vi "cluster_v30.vi"() -> ()   [LabVIEW 2009]
panel:
  in  "stop":bool
  out "Waveform Graph":dbl[](graph)=[1.340619718021982, -0.6009860791806715, -0.0535520537195435, -0.009542246662558042, -0.0025019088903811522, -0.0008379211165242679, -0.00033229836709205973, -0.0001491346742136413, -7.356383530775908e-05, -3.9094873850847784e-05, -2.2068047028342232e-05, -1.3092803157888074e-05, -8.099534476939332e-06, -5.1922069190088255e-06, -3.4322006682237186e-06, -2.3302383349082557e-06, -1.6196706723518948e-06, -1.1494371287666694e-06, -8.309954579634783e-07, -6.108580258527588e-07, -4.55831665919915e-07, -3.448134329849513e-07, -2.6409078418298253e-07, -2.0457511909595536e-07, -1.601327682386241e-07, -1.265552528967856e-07, -1.0091080697079654e-07, -8.112824407953131e-08, -6.572525460615341e-08, -5.362814023445084e-08, -4.40504248915006e-08, -3.6409976192492306e-08, -3.0271687098320935e-08, -2.5307355322970933e-08, -2.126728244966514e-08, -1.7959955674597112e-08, -1.5237366748646937e-08, -1.298430431167563e-08, -1.111047491101763e-08, -9.544656805788532e-09, -8.230327650586232e-09, -7.122369864548406e-09, -6.184570317657947e-09, -5.387709938770505e-09, -4.708094622012196e-09, -4.126418531238929e-09, -3.6268794239086245e-09, -3.196486252904076e-09, -2.824514347237582e-09, -2.5020745141628103e-09, -2.2217705646904717e-09, -1.9774258330295135e-09, -1.7638638017590042e-09, -1.5767313630623035e-09, -1.4123558343375948e-09, -1.2676288164209037e-09, -1.1399114899967575e-09, -1.0269571049789404e-09, -9.268473134588894e-10, -8.379396923335715e-10, -7.588243441645309e-10, -6.882878897192902e-10, -6.252834998757877e-10, -5.689058785471334e-10, -5.183703175936982e-10, -4.729951112841509e-10, -4.3218675095134046e-10, -3.9542742718203427e-10, -3.62264452710001e-10, -3.3230128846006416e-10, -3.051899112899401e-10, -2.8062430754683426e-10, -2.583349136860541e-10, -2.3808385554208473e-10, -2.196608627106848e-10, -2.0287975493853432e-10, -1.875754142597046e-10, -1.7360117053488108e-10, -1.6082653957780264e-10, -1.4913526262751594e-10, -1.3842360389551063e-10, -1.2859886956797358e-10, -1.1957811720650903e-10, -1.1128702915421086e-10, -1.0365892747200734e-10, -9.663391122896946e-11, -9.015809975347203e-11, -8.418296780510081e-11, -7.866476062047243e-11, -7.35639784779603e-11, -6.884492186502103e-11, -6.447528955753694e-11, -6.042582296675758e-11, -5.666999100392492e-11, -5.318371047881777e-11, -4.994509770578385e-11, -4.693424755573337e-11, -4.413303667883354e-11, -4.1524948041880945e-11, -3.909491428634135e-11]
  out "r":ext=0.91999999999999999947
  in  "eps":ext(slide)=9.449685534591195 scale=0.0..10.0
  in  "sig":ext(slide)=0.010056352459016394 scale=0.01..0.0105
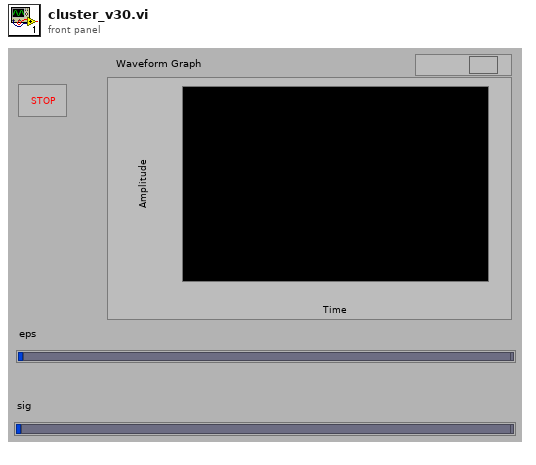
[diagram p1: front panel]
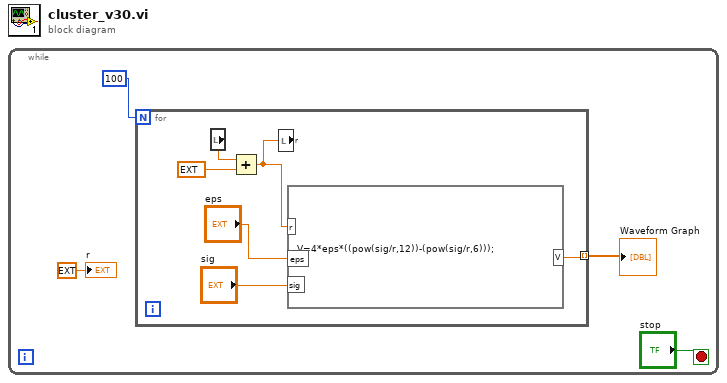
[diagram p0: block diagram]
diagram:
  n1 = while {
    stop <- "stop" stop-if-true
    n2 = for {
      N: 100 -> [_]
      tunnel: [w9] -> w2 mode=indexing
      n3 = local read "r"() -> (w10:ext)
      n4 = Add(x=w10, y=ext 0.01) -> (x+y=w5:ext)
      n5 = local write "r"(w5) -> ()
      n6 = formula code="V=4*eps*((pow(sig/r,12))-(pow(sig/r,6)));"("r"=w5, "eps"="eps", "sig"="sig") -> ("V"=w9:dbl)
    }
    "Waveform Graph" <- w2
    "r" <- ext 0.0 ("r")
  }
